vi "CC Obervation Generate Acquire Step.vi"(8 "error in (no error)":errorcluster, 9 "Dithering":string, 10 "Exposure":string="Auto", 11 "Object":string) -> (0 "error out":errorcluster, 3 "Acquire Step":T1={"Action"=enum."Acquire Images", "Data"=variant})   [LabVIEW 2024]
uses:
  typedefs/CC Script Step.ctl
  typedefs/CC enum Script Action.ctl
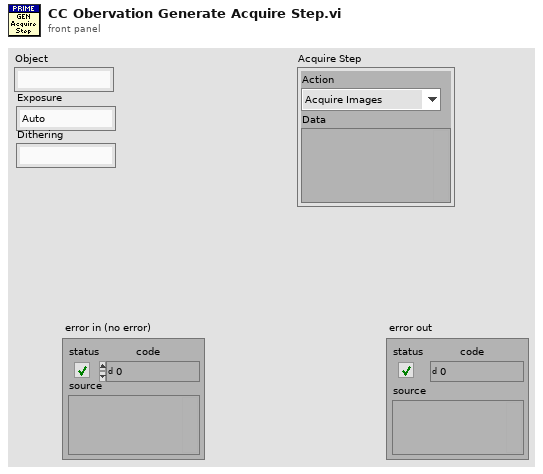
[diagram p1: front panel]
types:
  T1 = typedef "CC Script Step.ctl" = cluster{"Action":T2, "Data":variant}
  T2 = typedef "CC enum Script Action.ctl" = enum16{"Noop", "Define Object", "Define Exposure", "Define Dithering", "Acquire Images", "Set Filter Wheel", "Telescope Home", "Telescope Move", "Telescope RA DEC", "Focus Move Relative", "Focus Move Absolute", "Focus Set Home", "Macro", "Pause", "Ask User", "Define Random Dither", "CmdLine", "Outlet"}
  T3 = cluster{"Object":string, "Exposure":string, "Dithering":string}
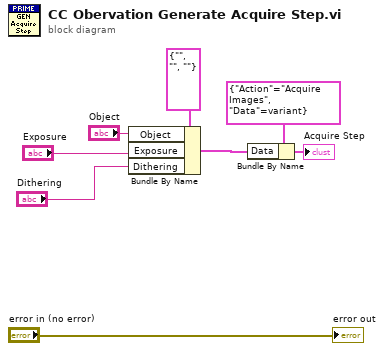
[diagram p0: block diagram]
diagram:
  n1 = Bundle By Name(cluster=T3 {"Object"="", "Exposure"="", "Dithering"=""} ("Acquire Parameters"), "Object"="Object", "Exposure"="Exposure", "Dithering"="Dithering") -> (w4:T3)
  n2 = Bundle By Name(cluster=T1 {"Action"=enum."Acquire Images", "Data"=variant} ("Cluster"), "Data"=w4) -> (→"Acquire Step":T1)
  "error out" <- "error in (no error)"
